vi "InitVI UI.vi"() -> ()   [LabVIEW 2015, in "Initialization.lvclass"]
uses:
  Initialization.lvclass
  <vilib>/NI/Configuration Framework/Node/NodeRef.ctl
  <vilib>/NI/Configuration Framework/Node/NISE_CEF_Node.lvclass
  <vilib>/NI/AMC/Message Queue.ctl
  <vilib>/NI/AMC/Message.ctl
  <vilib>/NI/Tools/Keyed Array/KeyedArray.ctl
  <vilib>/NI/Configuration Framework/Node/UserEventRef.ctl
  <vilib>/NI/Configuration Framework/Controls/EventCluster.ctl
  XML Controls/Execution Types.ctl
  Initialization.lvclass/Initialization.ctl
  Read Initialization VI Properties.vi
  Write Initialization VI Properties.vi
  <vilib>/NI/AMC/Create Single Message.vi
  <vilib>/NI/AMC/Update Message Routing Info.vi
  <vilib>/NI/AMC/Send Message.vi
  <vilib>/NI/AMC/AMC.lvlib
  Configuration Tool.lvlib
  <vilib>/NI/Tools/Keyed Array/Tools_KeyedArray.lvlib
  <vilib>/NI/Configuration Framework/NISE_CEF_TreeControl.lvlib
panel:
  in  "Position":enum16{"centered", "mouse pointer"}(ring)
  in  "Type":enum16{"Action", "VI"}(ring)
  in  "Execution":T1
  in  "Host Path to Initialization VI":path
  in  "user event":T2
  in  "main queue":T3
  in  "node ref":T4
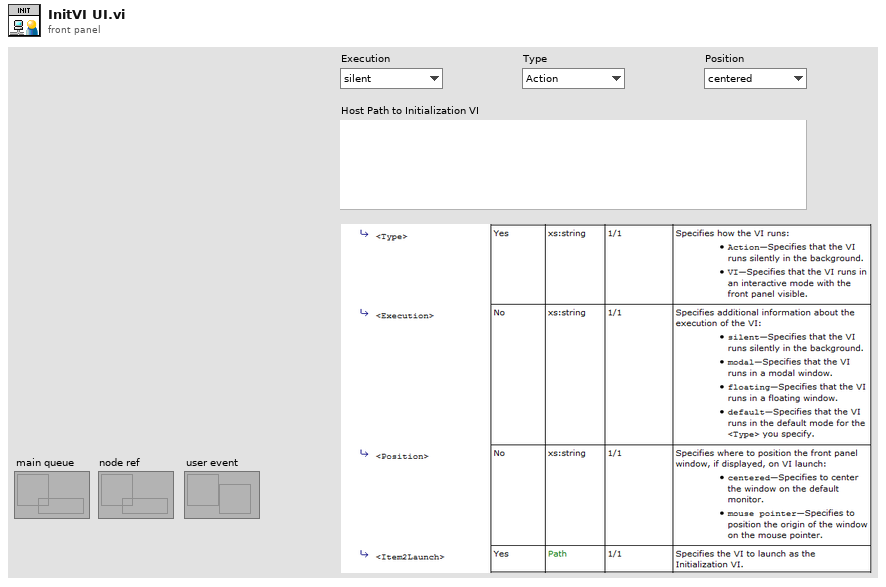
[diagram p1: front panel]
types:
  T1 = typedef "Configuration Tool.lvlib/Execution Types.ctl" = enum16{"silent", "modal", "floating", "default"}
  T2 = typedef "NISE_CEF_Node.lvclass/UserEventRef.ctl" = refnum<user-event>
  T3 = typedef "AMC.lvlib/Message Queue.ctl" = refnum<queue>
  T4 = typedef "NISE_CEF_Node.lvclass/NodeRef.ctl" = refnum<data-value>
  T5 = typedef "Initialization VI Properties.ctl" = cluster{"Execution":T6, "Path":T7, "Type":enum16{"Action", "VI"}, "Position":enum16{"centered", "mouse pointer"}}
  T6 = typedef "Execution Types.ctl" = enum16{"silent", "modal", "floating", "default"}
  T7 = typedef "Path Cluster.ctl" = cluster{"Path":path, "Path Type":enum16{"Absolute", "To Base", "To Common Doc Dir", "To Application Data Dir"}}
  T8 = enum16{"Absolute", "To Base", "To Common Doc Dir", "To Application Data Dir"}
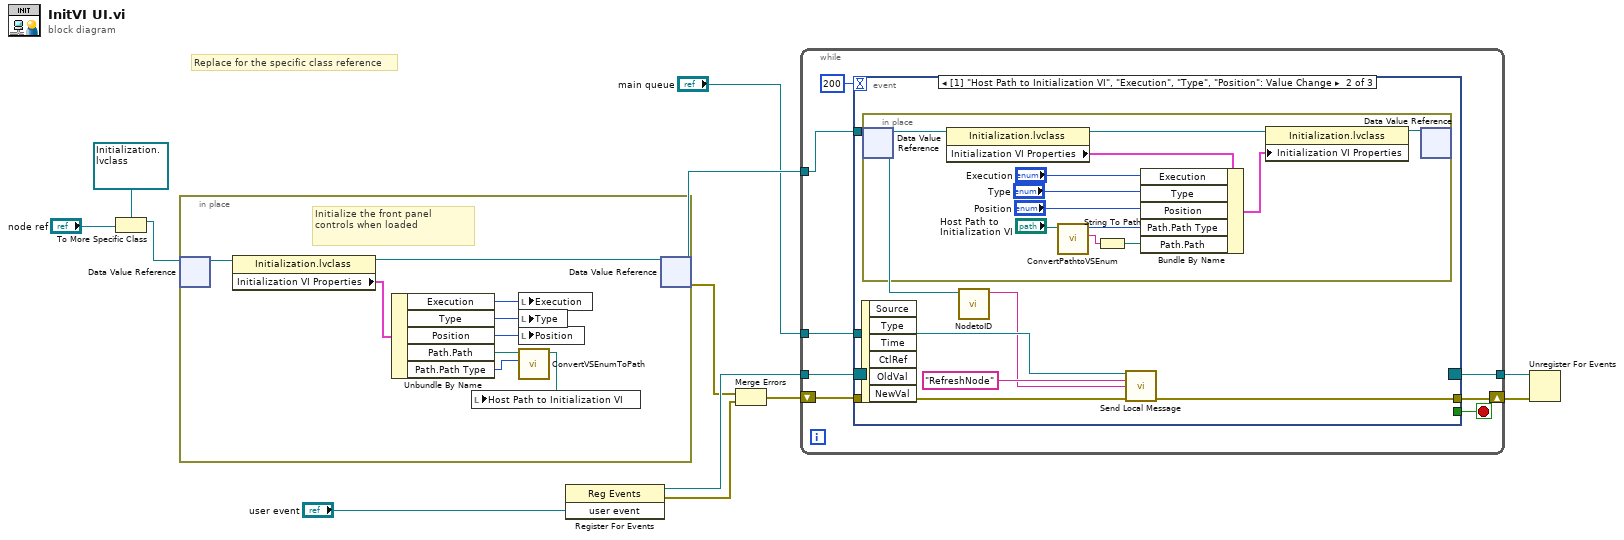
[diagram p0: block diagram]
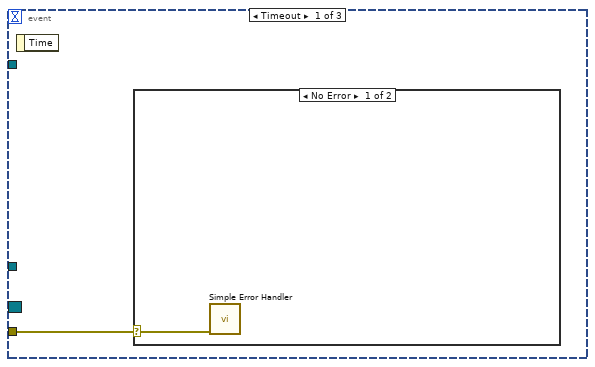
[diagram p2: hidden frame]
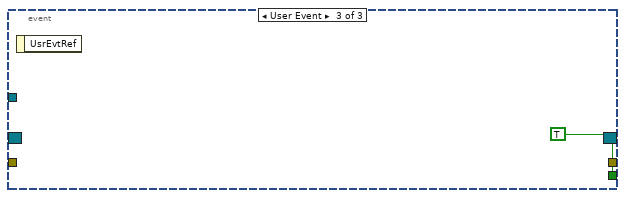
[diagram p4: hidden frame]
diagram:
  # "Replace for the specific class reference"
  n1 = To More Specific Class(target class=refnum<data-value> refnum ("data value reference"), reference="node ref") -> (specific class reference=w5:refnum<data-value>)  [unwired: 1 in, 1 out]
  n2 = in-place {
    # "Initialize the front panel controls when loaded"
    n3 = in-place-dvr #1(w5) -> (w21:refnum<class "Initialization.lvclass">)  [unwired: 1 out]
    n4 = property class="Initialization.lvclass"(reference=w21) -> (reference out=w20:refnum<class "Initialization.lvclass">, "Initialization VI Properties"=w19:T5)  [unwired: 1 in, 1 out]
    n5 = Unbundle By Name(w19) -> ("Execution"=w18:T6, "Type"=w17:enum16{"Action", "VI"}, "Position"=w16:enum16{"centered", "mouse pointer"}, "Path.Path"=w15:path, "Path.Path Type"=w14:T8)
    n6 = local write "Execution"(w18) -> ()
    n7 = local write "Type"(w17) -> ()
    n8 = local write "Position"(w16) -> ()
    n9 = call "ConvertVSEnumToPath.vi"("Source.Path Type"=w14, "Path In"=w15) -> ("appended path"=w13:path)  [unwired: 9 in]
    n10 = local write "Host Path to Initialization VI"(w13) -> ()
    n11 = in-place-dvr #1(w20) -> (w12:refnum<data-value>, w2:errorcluster)
  }
  n12 = register-events("user event") -> (reference out=w9:refnum<event-registration>, error out=w3:errorcluster)  [unwired: 2 in]
  n13 = Merge Errors(w2, w3) -> (w1:errorcluster)
  n14 = while {
    tunnel: w12 -> [w29]
    tunnel: "main queue" -> [w28]
    tunnel: w9 -> [w26]
    tunnel: [w25] -> w8
    shift-right: [w23] -> w7
    shift-left: w1 -> [w22]
    stop <- w24 stop-if-true
    n15 = event shown="[1] \"Host Path to Initialization VI\", \"Execution\", \"Type\", \"Position\": Value Change" {
      selector: w26 -> [_ _ _]
      dyn-events: [_ _ _] -> w25
      timeout: 200 -> [_ _ _]
      tunnel: w29 -> [_ w35 _]
      tunnel: w28 -> [_ w36 _]
      tunnel: [_ _ TRUE] -> w24
      tunnel: [_ w33 _] -> w23
      tunnel: w22 -> [w30 w32 _]
      event Timeout {
        n16 = event-data() -> ()  [unwired: 1 in, 1 out]
        n17 = case shown="No Error" w30 {
          selector: w30 -> [w31 _]
          frame No Error {
            n18 = call <vilib>:"Simple Error Handler.vi"("error in (no error)"=w31) -> ()  [unwired: 4 in, 5 out]
          }
          frame Error {
          }
        }
      }
      event "Host Path to Initialization VI", "Type", "Position": Value Change {
        n19 = event-data() -> ()  [unwired: 1 in, 6 out]
        n20 = in-place {
          n21 = in-place-dvr #2(w35) -> (w48:refnum<class "Initialization.lvclass">)  [unwired: 1 out]
          n22 = property class="Initialization.lvclass"(reference=w48) -> (reference out=w38:refnum<class "Initialization.lvclass">, "Initialization VI Properties"=w47:T5)  [unwired: 1 in, 1 out]
          n23 = call "ConvertPathtoVSEnum.vi"("Path In"="Host Path to Initialization VI") -> ("Remaining Path"=w46:string, "VS Enum Out"=w44:T8)  [unwired: 9 in]
          n24 = String To Path(string=w46) -> (path=w45:path)
          n25 = Bundle By Name(cluster=w47, "Execution"="Execution", "Type"="Type", "Position"="Position", "Path.Path Type"=w44, "Path.Path"=w45) -> (w39:T5)
          n26 = property class="Initialization.lvclass"(reference=w38, "Initialization VI Properties"=w39) -> (reference out=w49:refnum<class "Initialization.lvclass">)  [unwired: 1 in, 1 out]
          n27 = in-place-dvr #2(w49) -> ()  [unwired: 2 out]
        }
        n28 = call <vilib>:"NodetoID.vi"("node ref"=w35) -> ("ID"=w34:string)  [unwired: 9 in, 1 out]
        n29 = call <vilib>:"Send Local Message.vi"("message queue in"=w36, "message name"="RefreshNode" ("Message Name"), "message value"=w34, "error in"=w32) -> ("error out"=w33:errorcluster)  [unwired: 9 in, 2 out]
      }
      event User Event {
        n30 = event-data() -> ()  [unwired: 1 in, 1 out]
      }
    }
  }
  n31 = Unregister For Events(event registration refnum=w8, error in=w7) -> ()  [unwired: 1 out]
